vi "Keithley 24XX Read Single.vi"() -> ()   [LabVIEW 2019, in "Keithley 24XX.lvlib"]
doc: "This example shows how to configure a measurement and take a reading."
uses:
  Public/Data/Read (Single Point).vi
  Keithley 24XX.lvlib
panel:
  in  "Source Mode  (0: Voltage)":u16(ring) items=["Voltage", "Current"]
  in  "Compliance  Level (0.1)":dbl=0.1
  in  "Output Level (0)":dbl
  in  "Enable Resistance Auto Range (T:Enable)":bool=TRUE
  in  "Enable Current Auto Range (T:Enable)":bool=TRUE
  in  "Enable Voltage Auto Range (T:Enable)":bool=TRUE
  in  "Resistance Manual Range (1.0)":dbl=1.0
  in  "Current Manual Range (1.0)":dbl=1.0
  in  "Voltage Manual Range (1.0)":dbl=1.0
  out "Resistance":sgl
  out "Current":sgl
  out "Voltage":sgl
  in  "Serial Configuration":T1={"Baud Rate"=9600, "Parity"=0, "Data Bits"=8, "Stop Bits"=10, "Flow Control"=0} {"Flow Control" items=["None", "XON/XOFF", "RTS/CTS", "XON/XOFF & RTS/CTS", "DTR/DSR", "XON/XOFF & DTR/DSR"]; "Stop Bits" items=["1.0"=10, "1.5"=15, "2.0"=20]; "Data Bits" items=["7"=7, "8"=8]; "Parity" items=["None", "Odd", "Even", "Mark", "Space"]; "Baud Rate" items=["300"=300, "600"=600, "1200"=1200, "2400"=2400, "4800"=4800, "9600"=9600, "19200"=19200]}
  in  "VISA resource name":refnum<visa-resource-name>
  # "(c) 2006 National Instruments.  ALL RIGHTS RESERVED."
  # "(c) 2006 - 2015 National Instruments.  ALL RIGHTS RESERVED."
  # "Source Settings"
  # "Voltage Range Settings"
  # "Current Range Settings"
  # "Resistance Range Settings"
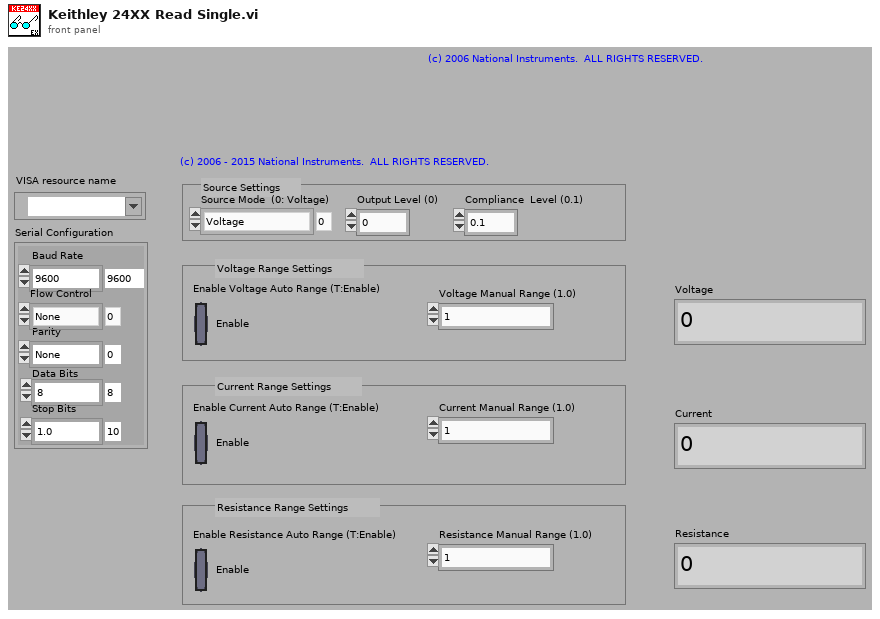
[diagram p1: front panel]
types:
  T1 = cluster{"Baud Rate":u32, "Parity":u16, "Data Bits":u16, "Stop Bits":u16, "Flow Control":u16}
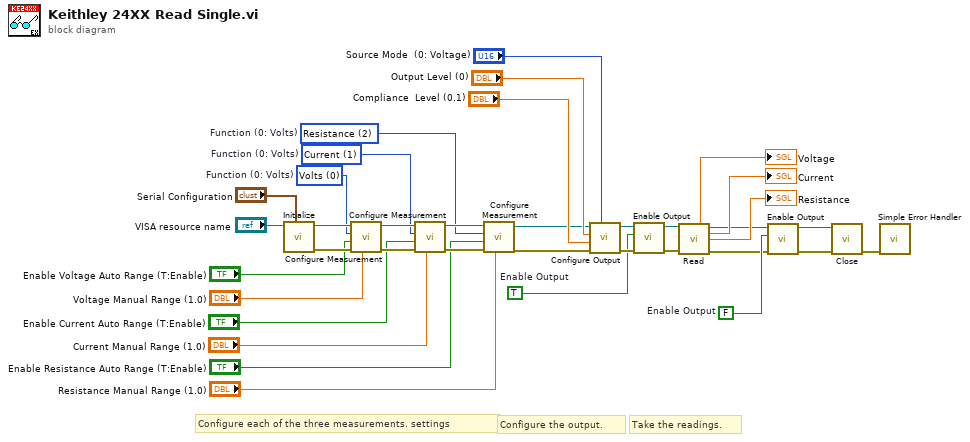
[diagram p0: block diagram]
diagram:
  w4 = TRUE  # Enable Output
  w15 = FALSE  # Enable Output
  w22 = u16 2 items=["Volts", "Current", "Resistance"]  # Function (0: Volts)
  w23 = u16 1 items=["Volts", "Current", "Resistance"]  # Function (0: Volts)
  w24 = u16 0 items=["Volts", "Current", "Resistance"]  # Function (0: Volts)
  # "Take the readings."
  # "Configure the output."
  # "Configure each of the three measurements. settings"
  n1 = call "Initialize.vi"("Serial Configuration"="Serial Configuration", "VISA resource name"="VISA resource name") -> ("error out"=w29:errorcluster, "VISA resource name out"=w30:refnum<visa-resource-name>)  [unwired: 8 in]
  n2 = call "Configure Measurement.vi"("Manual Range (1.0)"="Voltage Manual Range (1.0)", "error in (no error)"=w29, "Enable Auto Range (T:Enable)"="Enable Voltage Auto Range (T:Enable)", "Function (0: Volts)"=w24, "VISA resource name"=w30) -> ("error out"=w27:errorcluster, "VISA resource name out"=w28:refnum<visa-resource-name>)  [unwired: 5 in]
  n3 = call "Configure Measurement.vi"("Manual Range (1.0)"="Current Manual Range (1.0)", "error in (no error)"=w27, "Enable Auto Range (T:Enable)"="Enable Current Auto Range (T:Enable)", "Function (0: Volts)"=w23, "VISA resource name"=w28) -> ("error out"=w26:errorcluster, "VISA resource name out"=w25:refnum<visa-resource-name>)  [unwired: 5 in]
  n4 = call "Configure Measurement.vi"("Manual Range (1.0)"="Resistance Manual Range (1.0)", "error in (no error)"=w26, "Enable Auto Range (T:Enable)"="Enable Resistance Auto Range (T:Enable)", "Function (0: Volts)"=w22, "VISA resource name"=w25) -> ("error out"=w3:errorcluster, "VISA resource name out"=w2:refnum<visa-resource-name>)  [unwired: 5 in]
  n5 = call "Configure Output.vi"("Source Mode  (0: Voltage)"="Source Mode  (0: Voltage)", "error in (no error)"=w3, "Compliance  Level (0.1)"="Compliance  Level (0.1)", "Output Level (0)"="Output Level (0)", "VISA resource name"=w2) -> ("error out"=w5:errorcluster, "VISA resource name out"=w6:refnum<visa-resource-name>)  [unwired: 5 in]
  n6 = call "Enable Output.vi"("error in (no error)"=w5, "Enable Output (T: Enable)"=w4, "VISA resource name"=w6) -> ("error out"=w8:errorcluster, "VISA resource name out"=w7:refnum<visa-resource-name>)  [unwired: 7 in]
  n7 = call-poly "Read.vi"("VISA resource name"=w7, "error in (no error)"=w8) -> ("Voltage"=→"Voltage":sgl, "VISA resource name out"=w9:refnum<visa-resource-name>, "Current"=→"Current":sgl, "Resistance"=→"Resistance":sgl, "error out"=w10:errorcluster)  [unwired: 7 in, 2 out]
  n8 = call "Enable Output.vi"("error in (no error)"=w10, "Enable Output (T: Enable)"=w15, "VISA resource name"=w9) -> ("error out"=w11:errorcluster, "VISA resource name out"=w12:refnum<visa-resource-name>)  [unwired: 7 in]
  n9 = call "Close.vi"("error in (no error)"=w11, "VISA resource name"=w12) -> ("error out"=w36:errorcluster)  [unwired: 9 in]
  n10 = call <vilib>:"Simple Error Handler.vi"("error in (no error)"=w36) -> ()  [unwired: 4 in, 5 out]
